vi "Doppler_Spectra.vi"(0 "Thresholds":T1={"Spec Ratio Threshold"=0.0, "V Threshold"=0.0, "Power Threshold"=0.0, "RF Threshold"=10000.0}, 5 "slow time":csg[](array[numeric]), 7 "Doppler Params":T2={"Dopp Filter Order"=2, "Window length"=64, "Window Increment"=64, "Start f"=0.05, "lDoppler cutouff"=10.0, "FFT Length"=512, "SlowTime (Hz)"=100.0} {"Start f" format="%0.3f"; "SlowTime (Hz)" format="%0.1f"; "lDoppler cutouff" format="%0.3f"}, 13 "Header In":T3 {"Compression Parameters"."% taper" min=50 max=1000 format="%.2f"; "Compression Parameters"."F2 (MHz)" format="%.3f"; "Compression Parameters"."F1 (MHz)" format="%.3f"; "Scan Settings"."prf (kHz)" format="%.2f"; "Therapy Parameters"."Therapy amplitude (mV)" min=50 max=1000 format="%.2f"; "Therapy Parameters"."Time on (s)" format="%.3f"; "Therapy Parameters"."Theraputic Freq (MHz)" format="%.3f"; "Patient Info"."Race" items=["Am Ind or Alaska", "Asian", "Hawaiian, Pac Isl", "Black or Afr Amer", "White", "more than one race", "unknown"]; "Patient Info"."Ethnicty 2" items=["Hispanic", "Non-Hispanic", "unknown"]; "Patient Info"."LOS" items=["1", "2", "3", "4", "5"]; "Patient Info"."PSA" format="%.1f"; "Scan Info"."delay" format="%.2f"; "Scan Info"."pivot distance" format="%.2f"; "Scan Info"."sector scan angle" format="%.2f"; "Tranducer Info"."bandwidth" format="%.2f"; "Tranducer Info"."center freq" format="%.2f"; "Tranducer Info"."start freq" format="%.2f"}) -> (1 "PowerRaw":sgl[][](array[numeric]), 2 "Mean Power":sgl[](array[numeric]), 3 "phase (old Fd AC)":sgl[](array[numeric]), 4 "Max indexs":i32[](array[numeric]), 6 "Total Power (dB)":sgl[](array[numeric]), 8 "Mag Dop Spec":dbl[][](graph), 10 "Slow time sampling":dbl, 12 "Unwrapped Phase":dbl[](array[numeric]), 14 "theta":dbl[](array[numeric]), 15 "Spec P Ratio":sgl[](array[numeric]))   [LabVIEW 2022 SP3]
uses:
  ViewData/-ReadEye/Header.ctl
  DopplerParams.ctl
  DopThresholds.ctl
  <vilib>/Analysis/2dsp.llb/Complex FFT.vi
  <vilib>/Analysis/8numeric.llb/1D Numeric Integration.vi
  <vilib>/Analysis/4window.llb/Hamming Window (CDB).vi
  <vilib>/Analysis/baseanly.llb/Mean (DBL).vi
  <vilib>/Analysis/4window.llb/AllCosWindow (CDB).vi
  <vilib>/Analysis/NI_AALPro.lvlib
  <vilib>/Analysis/NI_AALBase.lvlib
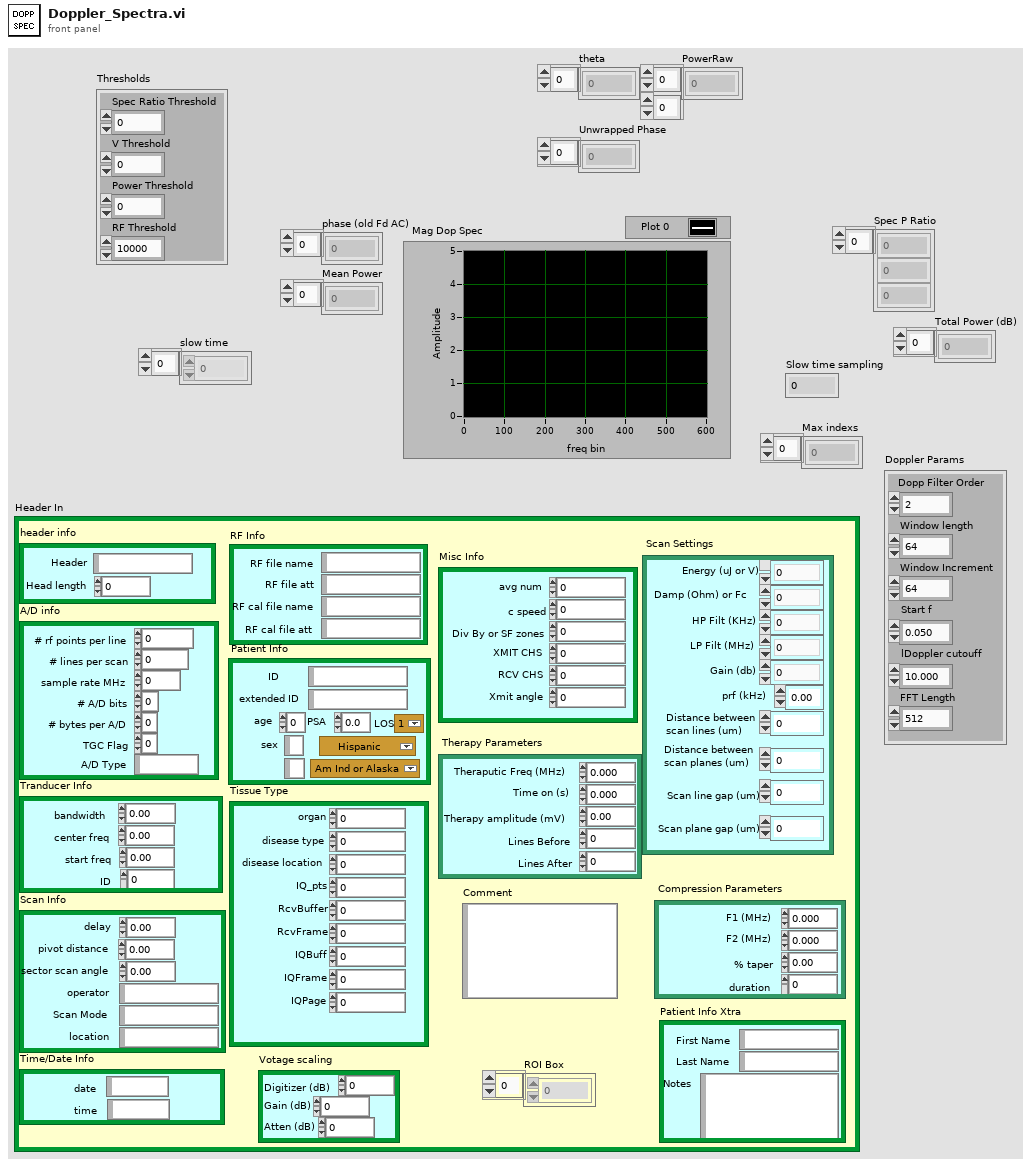
[diagram p1: front panel]
types:
  T1 = typedef "DopThresholds.ctl" = cluster{"Spec Ratio Threshold":dbl, "V Threshold":dbl, "Power Threshold":dbl, "RF Threshold":dbl}
  T2 = typedef "DopplerParams.ctl" = cluster{"Dopp Filter Order":i32, "Window length":i32, "Window Increment":i32, "Start f":dbl, "lDoppler cutouff":dbl, "FFT Length":i32, "SlowTime (Hz)":dbl}
  T3 = typedef "Header.ctl" = cluster{"header info":cluster{"Header":string, "Head length":i16}, "A/D info":cluster{"# rf points per line":u16, "# lines per scan":u16, "sample rate MHz":u16, "# A/D bits":i16, "# bytes per A/D":u16, "TGC Flag":u16, "A/D Type":string}, "Tranducer Info":cluster{"bandwidth":sgl, "center freq":sgl, "start freq":sgl, "ID":i32}, "Scan Info":cluster{"delay":sgl, "pivot distance":sgl, "sector scan angle":sgl, "operator":string, "Scan Mode":string, "location":string}, "Time/Date Info":cluster{"date":string, "time":string}, "RF Info":cluster{"RF file name":string, "RF file att":string, "RF cal file name":string, "RF cal file att":string}, "Patient Info":cluster{"ID":string, "extended ID":string, "age":u16, "sex":string, "previously\nscanned":string, "PSA":sgl, "LOS":u8, "Ethnicty 2":u8, "Race":u8}, "Tissue Type":cluster{"organ":i16, "disease type":i16, "disease location":i16, "IQ_pts":u16, "RcvBuffer":u8, "RcvFrame":u16, "IQBuff":u8, "IQFrame":u16, "IQPage":u8}, "Votage scaling":cluster{"Digitizer (dB)":sgl, "Gain (dB)":sgl, "Atten (dB)":sgl}, "Comment":string, "Misc Info":cluster{"avg num":u16, "c speed":i16, "Div By or SF zones":i16, "XMIT CHS":u8, "RCV CHS":u8, "Xmit angle":sgl}, "Therapy Parameters":cluster{"Theraputic Freq (MHz)":sgl, "Time on (s)":sgl, "Therapy amplitude (mV)":sgl, "Lines Before":u16, "Lines After":u16}, "Scan Settings":cluster{"Energy (uJ or V)":u8, "Damp (Ohm) or Fc":u8, "HP Filt (KHz)":u8, "LP Filt (MHz)":u8, "Gain (db)":u8, "prf (kHz)":sgl, "Distance between\nscan lines (um)":u16, "Distance between\nscan planes (um)":u16, "Scan line gap (um)":sgl, "Scan plane gap (um)":sgl}, "Compression Parameters":cluster{"F1 (MHz)":sgl, "F2 (MHz)":sgl, "% taper":sgl, "duration":sgl}, "Patient Info Xtra":cluster{"First Name":string, "Last Name":string, "Notes":string}, "ROI Box":u16[]}
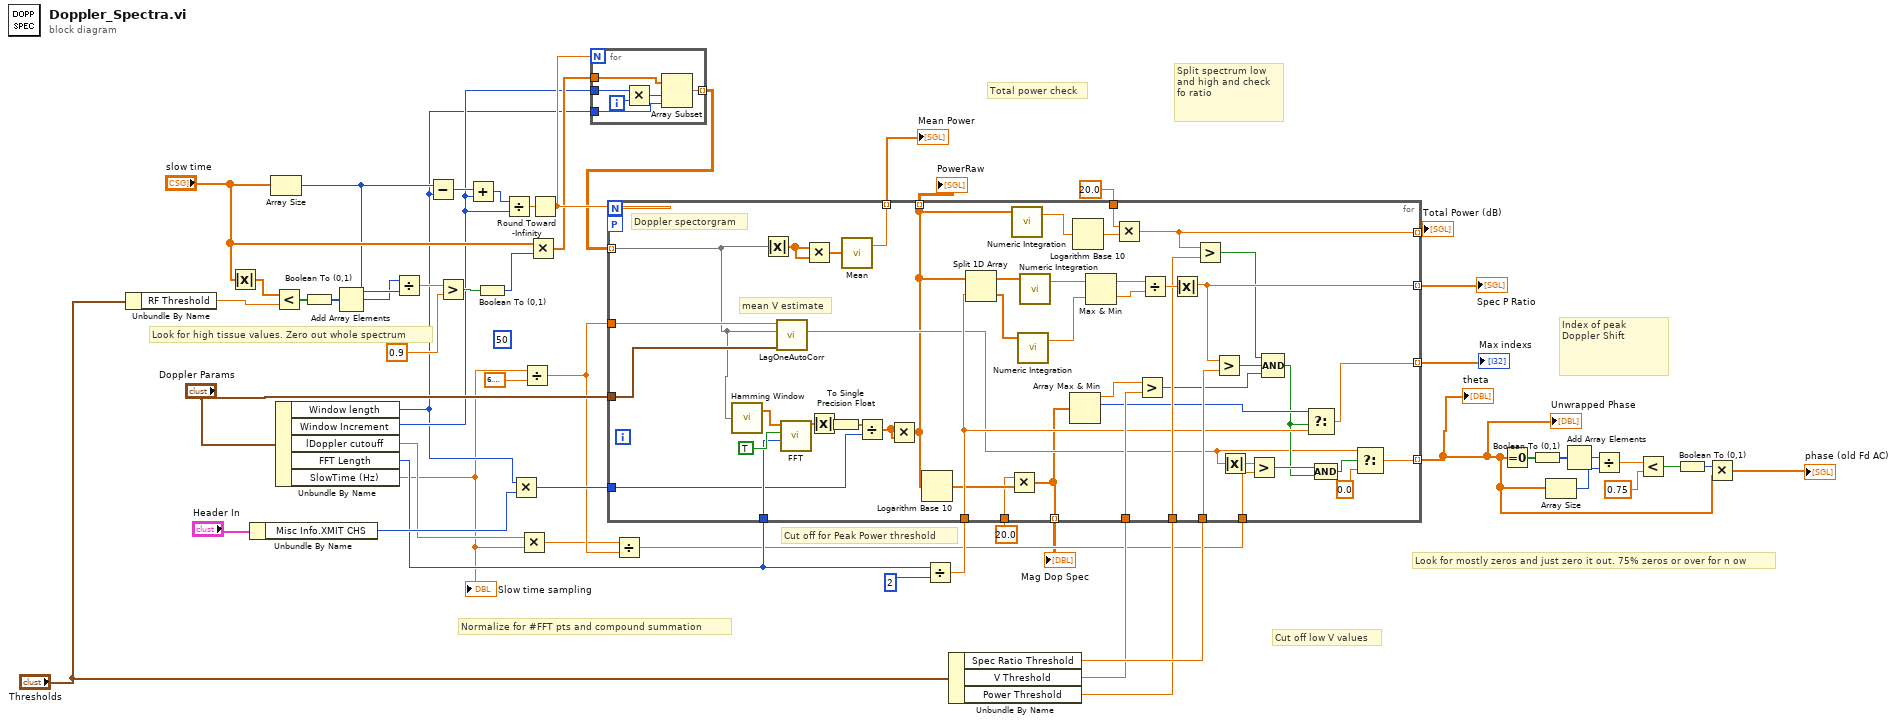
[diagram p0: block diagram]
diagram:
  (unwired) i16 50 ("y")
  # "Index of peak Doppler Shift"
  # "Cut off for Peak Power threshold"
  # "Total power check"
  # "Cut off low V values"
  # "Split spectrum low and high and check fo ratio"
  # "Look for mostly zeros and just zero it out. 75% zeros or over for n ow"
  # "Look for high tissue values. Zero out whole spectrum"
  # "Normalize for #FFT pts and compound summation"
  n1 = Unbundle By Name("Thresholds") -> ("RF Threshold"=w33:dbl)
  n2 = Absolute Value(x="slow time") -> (abs(x)=w32:sgl[])
  n3 = Unbundle By Name("Header In") -> ("Misc Info.XMIT CHS"=w44:u8)
  n4 = Array Size(array="slow time") -> (size(s)=w30:i32)
  n5 = Less?(x=w32, y=w33) -> (x < y?=w35:bool[])
  n6 = Unbundle By Name("Doppler Params") -> ("Window length"=w5:i32, "Window Increment"=w7:i32, "lDoppler cutouff"=w4:dbl, "FFT Length"=w38:i32, "SlowTime (Hz)"=w2:dbl)
  "Slow time sampling" <- w2
  n7 = Boolean To (0,1)(Boolean=w35) -> (0, 1=w34:i16[])
  n8 = Add Array Elements(numeric array=w34) -> (sum=w29:i16)
  n9 = Divide(x=w29, y=w30) -> (x/y=w28:dbl)
  n10 = Subtract(x=w30, y=w5) -> (x-y=w53:i32)
  n11 = Greater?(x=w28, y=0.9) -> (0:w26:bool)
  n12 = Add(x=w53, y=w7) -> (x+y=w54:i32)
  n13 = Boolean To (0,1)(Boolean=w26) -> (0, 1=w25:i16)
  n14 = Divide(x=w54, y=w7) -> (x/y=w52:dbl)
  n15 = Multiply(x=w5, y=w44) -> (x*y=w43:i32)
  n16 = Multiply(x=w4, y=w2) -> (x*y=w3:dbl)
  n17 = Divide(x=w2, y=6.283185307179586) -> (x/y=w16:dbl)
  n18 = Multiply(x="slow time", y=w25) -> (x*y=w8:csg[])
  n19 = Round Toward -Infinity(1:w52) -> (0:w9:dbl)
  n20 = for {
    N: w9 -> [_]
    tunnel: w8 -> [w59]
    tunnel: w7 -> [w58]
    tunnel: [w56] -> w6 mode=indexing
    tunnel: w5 -> [w55]
    i -> [w57]
    n21 = Multiply(x=w58, y=w57) -> (x*y=w60:i32)
    n22 = Array Subset(array=w59, index=w60, length=w55) -> (w56:csg[])
  }
  n23 = Divide(x=w3, y=w16) -> (x/y=w15:dbl)
  n24 = Divide(x=w38, y=2) -> (x/y=w48:dbl)
  n25 = Unbundle By Name("Thresholds") -> ("Spec Ratio Threshold"=w47:dbl, "V Threshold"=w42:dbl, "Power Threshold"=w46:dbl)
  n26 = for {
    N: w9 -> [_]
    tunnel: [w87] -> w51 mode=indexing
    tunnel: w6 -> [w62] mode=indexing
    tunnel: w42 -> [w105]
    tunnel: w48 -> [w88]
    tunnel: [w99] -> w50 mode=indexing
    tunnel: w38 -> [w101]
    tunnel: w47 -> [w98]
    tunnel: [w64] -> w41 mode=indexing
    tunnel: w46 -> [w92]
    tunnel: w16 -> [w86]
    tunnel: [w72] -> w13 mode=indexing
    tunnel: w43 -> [w84]
    tunnel: w15 -> [w81]
    tunnel: [w78] -> w40 mode=indexing
    tunnel: "Doppler Params" -> [w74]
    tunnel: [w68] -> w12 mode=indexing
    tunnel: 20.0 ("x/y") -> [w69]
    tunnel: 20.0 ("x/y") -> [w63]
    workers-P: _ -> [_]
    tunnel: [w61] -> w1 mode=indexing
    # "mean V estimate"
    # "Doppler spectorgram"
    n27 = call-poly <vilib>:"Hamming Window.vi"("X"=w62) -> ("Windowed X"=w93:cdb[])  [unwired: 1 out]
    n28 = Absolute Value(x=w62) -> (abs(x)=w67:sgl[])
    n29 = call "LagOneAutoCorr.vi"("Doppler Params"=w74, "slow time"=w62, "angular Scalar"=w86) -> ("phase"=w73:dbl)  [unwired: 7 in, 1 out]
    n30 = call-poly <vilib>:"FFT.vi"("FFT size"=w101, "shift?"=TRUE, "X"=w93) -> ("FFT {X}"=w106:cdb[])  [unwired: 7 in, 1 out]
    n31 = Multiply(x=w67, y=w67) -> (x*y=w77:sgl[])
    n32 = Absolute Value(x=w106) -> (abs(x)=w100:dbl[])
    n33 = To Single Precision Float(number=w100) -> (single precision float=w75:sgl[])
    n34 = call-poly <vilib>:"Mean.vi"("X"=w77) -> ("mean"=w78:dbl)  [unwired: 1 out]
    n35 = Divide(x=w75, y=w84) -> (x/y=w71:sgl[])
    n36 = Multiply(x=w71, y=w71) -> (x*y=w61:sgl[])
    n37 = Logarithm Base 10(1:w61) -> (0:w70:sgl[])
    n38 = Split 1D Array(array=w61, index=w88) -> (first subarray=w103:sgl[], second subarray=w104:sgl[])
    n39 = Multiply(x=w69, y=w70) -> (x*y=w68:dbl[])
    n40 = call-poly <vilib>:"Numeric Integration.vi"("Input Array"=w61) -> ("result"=w65:dbl)  [unwired: 2 in, 1 out]
    n41 = call-poly <vilib>:"Numeric Integration.vi"("Input Array"=w104) -> ("result"=w96:dbl)  [unwired: 2 in, 1 out]
    n42 = call-poly <vilib>:"Numeric Integration.vi"("Input Array"=w103) -> ("result"=w97:dbl)  [unwired: 2 in, 1 out]
    n43 = Array Max & Min(array=w68) -> (max value=w107:dbl, max index (indices)=w89:i32)  [unwired: 2 out]
    n44 = Logarithm Base 10(1:w65) -> (0:w66:dbl)
    n45 = Max & Min(x=w97, y=w96) -> (max(x,y)=w95:dbl, min(x,y)=w94:dbl)
    n46 = Multiply(x=w63, y=w66) -> (x*y=w64:dbl)
    n47 = Greater?(x=w107, y=w105) -> (0:w85:bool)
    n48 = Divide(x=w95, y=w94) -> (x/y=w102:dbl)
    n49 = Absolute Value(x=w102) -> (abs(x)=w99:dbl)
    n50 = Greater?(x=w64, y=w92) -> (0:w91:bool)
    n51 = Greater?(x=w99, y=w98) -> (0:w90:bool)
    n52 = Absolute Value(x=w73) -> (abs(x)=w79:dbl)
    n53 = Greater?(x=w79, y=w81) -> (0:w83:bool)
    n54 = Compound Arithmetic op=AND(w91, w90, w85) -> (w80:bool)
    n55 = Select(t=w89, s=w80, f=w88) -> (s? t:f=w87:dbl)
    n56 = Compound Arithmetic op=AND(w83, w80) -> (w82:bool)
    n57 = Select(t=w73, s=w82, f=0.0 ("t")) -> (s? t:f=w72:dbl)
  }
  "Max indexs" <- w51
  "Mag Dop Spec" <- w12
  "Spec P Ratio" <- w50
  "Total Power (dB)" <- w41
  "Mean Power" <- w40
  "theta" <- w13
  "Unwrapped Phase" <- w13
  "PowerRaw" <- w1
  n58 = Equal To 0?(x=w13) -> (x = 0?=w24:bool[])
  n59 = Boolean To (0,1)(Boolean=w24) -> (0, 1=w23:i16[])
  n60 = Array Size(array=w13) -> (size(s)=w18:i32)
  n61 = Add Array Elements(numeric array=w23) -> (sum=w22:i16)
  n62 = Divide(x=w22, y=w18) -> (x/y=w21:dbl)
  n63 = Less?(x=w21, y=0.75) -> (x < y?=w19:bool)
  n64 = Boolean To (0,1)(Boolean=w19) -> (0, 1=w17:i16)
  n65 = Multiply(x=w17, y=w13) -> (x*y=→"phase (old Fd AC)":dbl[])
